vi "State Manager.vi"(1 "Previous State":T1, 2 "Current State":T1, 3 "Event":T2=enum."Green Tape Crossed") -> (0 "Next State":T1=enum."Stagger Stop")   [LabVIEW 2017]
uses:
  Event.ctl
  State.ctl
panel:
  out "Course Stage":i32=3
  # "The Algorithm:\n\nInit: [Wait]\n\nState: [Wait]\nWhen: {Start} --> [Follow Wall: 1]\n\n~~~ NOT IMPLEMENTED ~~~\nState: [<state>]\nWhen: <state> != [Zig Zag Hazard] & {Tape Edge Too Close} --> [Recenter: <state>]\nWhen: <state> != [Zig Zag Hazard] & {Wall Too Close} --> [Recenter: <state>]\n~~~~~~~~~~~~~~~~~~~~\n\nState: [Recenter: <prev_state>]\nWhen: {Centered} --> <prev_state>\n\nState: [Follow Wall: <stage>]\nWhen: {Black & Yellow Tape} --> [Zig Zag: <stage>, 1]\nWhen: {Red Tape Touched} --> [Ramp: <stage>]\nWhen: <stage> = 4 & {Rough Terrain Touched} --> [Cross Rough Terrain: <stage>]\nWhen: <stage> = 6 & {Green Tape Crossed} --> [Stagger Stop]\nWhen: {Black Tape Crossed} --> [Follow Wall: <stage> + 1]\n\nState: [Zig Zag: <stage>, <zig_zag_num>]\nWhen: <zig_zag_num> = 4 --> [Follow Wall: <stage>]\nWhen: {Tape Edge Too Close} | {Wall Too Close}\n    --> [Zig Zag: <stage>, <zig_zag_num> + 1]\n\nState: [Ramp: <stage>]\nWhen: {Ramp Passed} --> [Follow Wall: <stage>]\n\nState: [Cross Rough Terrain: <stage>]\nWhen: {Rough Terrain Passed} --> [Follow Wall: <stage>]\n\nState: [Stagger Stop]\nWhen: {Stop Button Pressed} --> [Wait]\nWhen: {End Zone Wait Timed Out} --> [Recenter]"
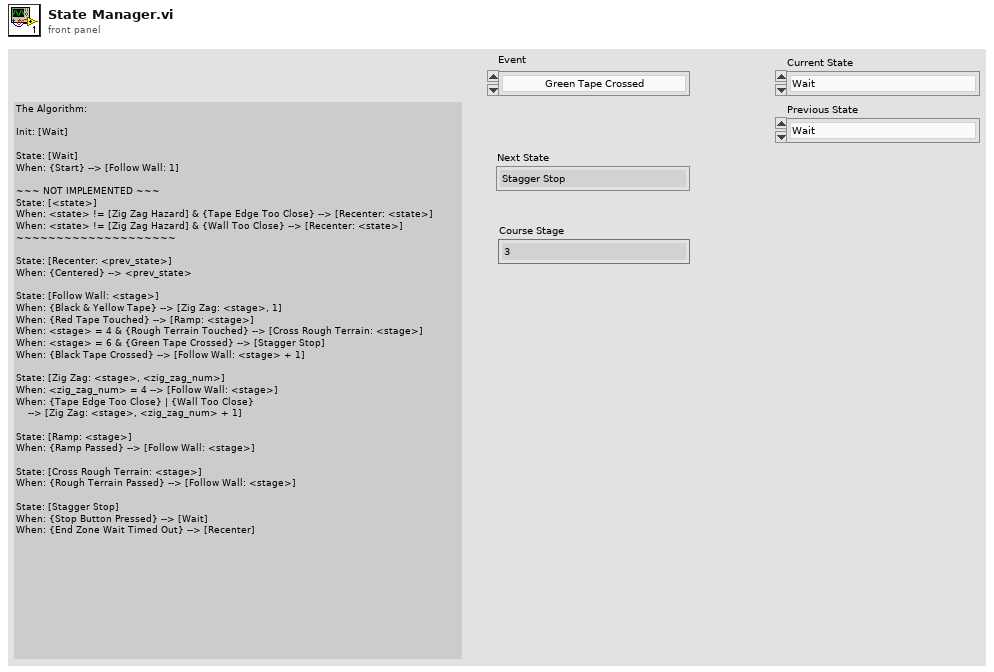
[diagram p1: front panel]
types:
  T1 = typedef "State.ctl" = enum16{"Wait", "Recenter", "Follow Wall", "Zig Zag", "Ramp", "Cross Rough Terrain", "Stagger Stop", "Obstacle Avoidance"}
  T2 = typedef "Event.ctl" = enum16{"None", "Zig Zag Finished", "Start Obstacle Avoidance", "Start Button Pressed", "Black & Yellow Tape Touched", "Black & Yellow Tape Passed", "Green Tape Crossed", "Red Tape Touched", "Rough Terrain Touched", "Black Tape Crossed", "Tape Edge Too Close", "Wall Too Close", "Rough Terrain Passed", "Ramp Passed", "Stop Button Pressed", "Recentered", "End Zone Wait Timed Out"}
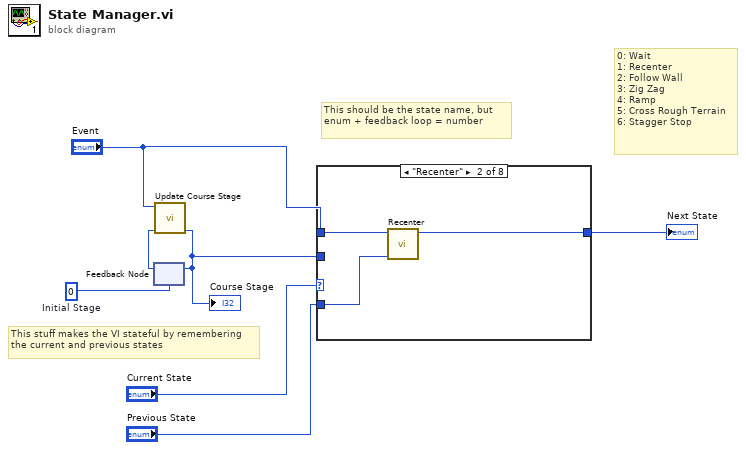
[diagram p0: block diagram]
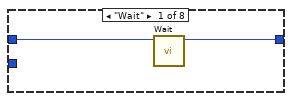
[diagram p2: hidden frame]
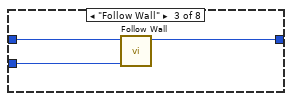
[diagram p3: hidden frame]
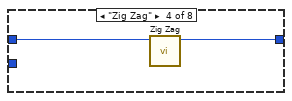
[diagram p4: hidden frame]
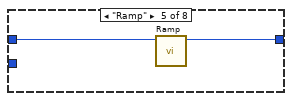
[diagram p5: hidden frame]
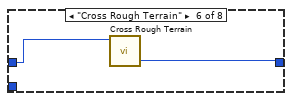
[diagram p6: hidden frame]
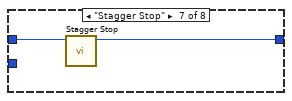
[diagram p7: hidden frame]
diagram:
  w6 = 0  # Initial Stage
  # "0: Wait\n1: Recenter\n2: Follow Wall\n3: Zig Zag\n4: Ramp\n5: Cross Rough Terrain\n6: Stagger Stop"
  # "This stuff makes the VI stateful by remembering the current and previous states"
  # "This should be the state name, but enum + feedback loop = number"
  n1 = feedback #1(w6) -> (w5:i32)
  n2 = call "Update Course Stage.vi"("Course Stage"=w5, "Event"="Event") -> ("New Course Stage"=w3:i8)  [unwired: 9 in]
  "Course Stage" <- w3
  n3 = feedback-in #1(w3) -> ()
  n4 = case shown="\"Recenter\"" "Current State" {
    selector: "Current State" -> [_ _ _ _ _ _ _ w24]
    tunnel: [w9 w11 w14 w16 w18 w21 w22 w24] -> w7
    tunnel: "Event" -> [w8 w12 w15 w17 w19 w20 w23 _]
    tunnel: "Previous State" -> [_ w10 _ _ _ _ _ _]
    tunnel: w3 -> [_ _ w13 _ _ _ _ _]
    frame "Wait" {
      n5 = call "Wait.vi"("Event"=w8) -> ("Next State"=w9:u16)  [unwired: 10 in]
    }
    frame "Recenter" {
      n6 = call "Recenter.vi"("Previous State"=w10, "Event"=w12) -> ("Next State"=w11:u16)  [unwired: 9 in]
    }
    frame "Follow Wall" {
      n7 = call "Follow Wall.vi"("Course Stage"=w13, "Event"=w15) -> ("Next State"=w14:u16)  [unwired: 9 in]
    }
    frame "Zig Zag" {
      n8 = call "Zig Zag.vi"("Event"=w17) -> ("Next State"=w16:u16)  [unwired: 10 in]
    }
    frame "Ramp" {
      n9 = call "Ramp.vi"("Event"=w19) -> ("Next State"=w18:u16)  [unwired: 10 in]
    }
    frame "Cross Rough Terrain" {
      n10 = call "Cross Rough Terrain.vi"("Event"=w20) -> ("Next State"=w21:u16)  [unwired: 10 in]
    }
    frame "Stagger Stop" {
      n11 = call "Stagger Stop.vi"("Event"=w23) -> ("Next State"=w22:u16)  [unwired: 10 in]
    }
    frame Default {
    }
  }
  "Next State" <- w7
